vi "LookForMultEOF.vi"(1 "Reply EOF":string) -> (0 "Array":string[](array[string]))   [LabVIEW 2012]
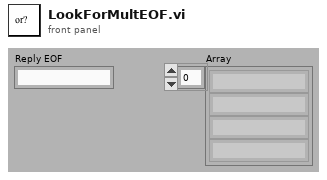
[diagram p1: front panel]
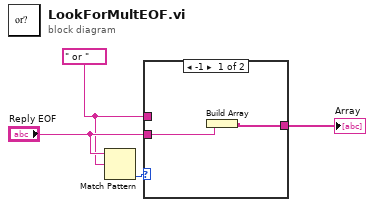
[diagram p0: block diagram]
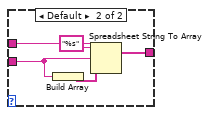
[diagram p2: hidden frame]
diagram:
  w2 = " or " ("delimiter (Tab)")
  n1 = Match Pattern(string="Reply EOF", regular expression=w2) -> (offset past match=w1:i32)  [unwired: 1 in, 3 out]
  n2 = case shown="-1" w1 {
    tunnel: [w5 w9] -> w4
    tunnel: "Reply EOF" -> [w6 w8]
    tunnel: w2 -> [_ w7]
    frame -1 {
      n3 = Build Array(w6) -> (w5:string[])
    }
    frame Default {
      n4 = Build Array(w8) -> (w10:string[])
      n5 = Spreadsheet String To Array(delimiter (Tab)=w7, format string="%s", spreadsheet string=w8, array type (2D Dbl)=w10) -> (array=w9:string[])
    }
  }
  "Array" <- w4
